vi "Read RemotePort.vi"(8 "error in (no error)":errorcluster, 11 "TrigBoxINIFileClass in":refnum<class "TrigBoxINIFileClass.lvclass">) -> (0 "error out":errorcluster, 2 "RemotePort":u16, 3 "TrigBoxINIFileClass out":refnum<class "TrigBoxINIFileClass.lvclass">)   [LabVIEW 2013, in "TrigBoxINIFileClass.lvclass"]
uses:
  TrigBoxINIFileClass.lvclass
  TrigBoxINIFileClass.lvclass/TrigBoxINIFileClass.ctl
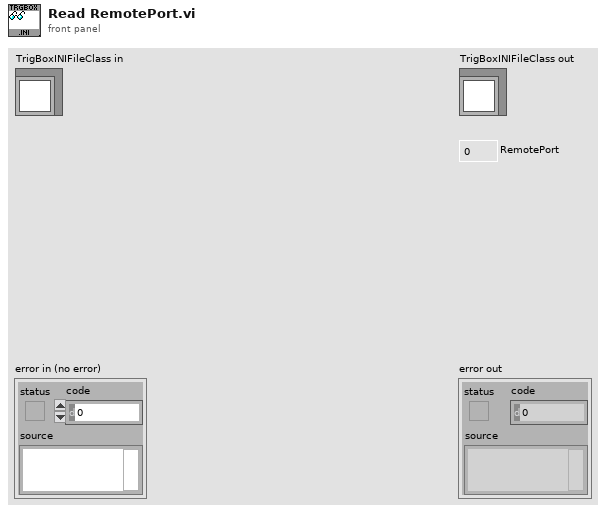
[diagram p1: front panel]
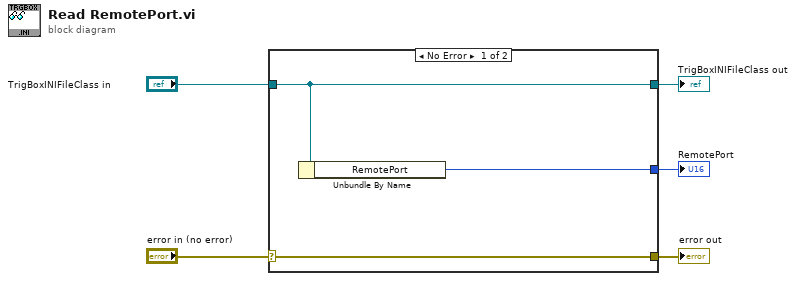
[diagram p0: block diagram]
diagram:
  n1 = case shown="No Error" "error in (no error)" {
    selector: "error in (no error)" -> [w8 w9]
    tunnel: [w8 w9] -> w4
    tunnel: [w7 w10] -> w2
    tunnel: "TrigBoxINIFileClass in" -> [w7 w10]
    tunnel: [w6 _] -> w1
    frame No Error {
      n2 = Unbundle By Name(w7) -> ("RemotePort"=w6:u16)
    }
    frame Error {
    }
  }
  "error out" <- w4
  "TrigBoxINIFileClass out" <- w2
  "RemotePort" <- w1
